vi "Download Bitfile.vi"(8 "error in (no error)":errorcluster, 10 "Port data.RIO device address":u16, 11 "path":path) -> (0 "error out":errorcluster, 5 "FPGA Session":u32)   [LabVIEW 2015, in "Diagnostics Addon Engine.lvlib"]
uses:
  Diagnostics Addon Engine.lvlib
  <vilib>/rvi/Utilities/XML/nirviXML_GetValue_String.vi
  NiFpga.dll
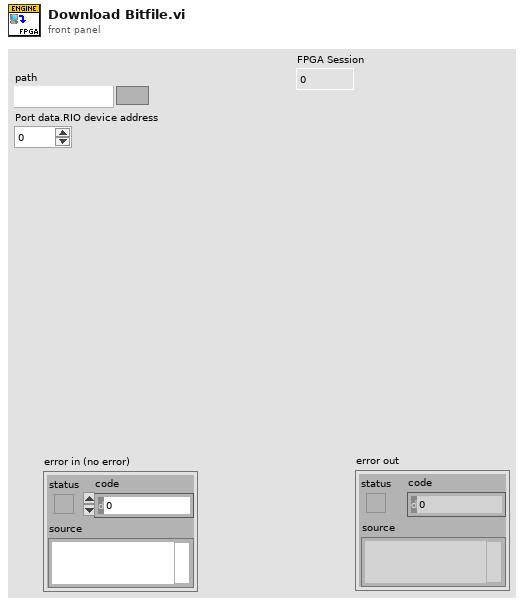
[diagram p1: front panel]
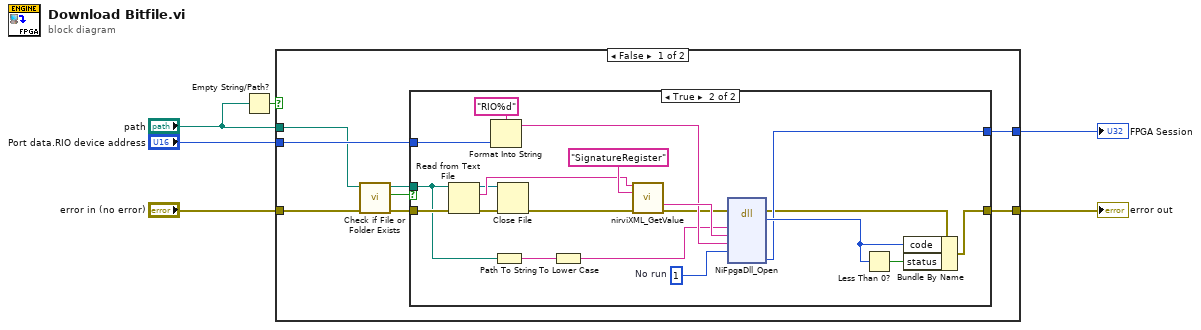
[diagram p0: block diagram]
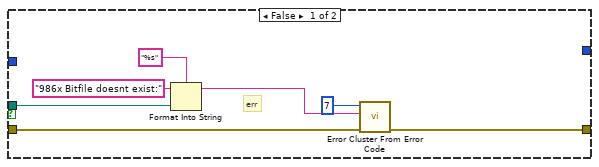
[diagram p2: hidden frame]
diagram:
  n1 = Empty String/Path?(string/path="path") -> (empty?=w3:bool)
  n2 = case shown="False" w3 {
    tunnel: "error in (no error)" -> [w13 w42]
    tunnel: [w14 w42] -> w5
    tunnel: "path" -> [w7 _]
    tunnel: "Port data.RIO device address" -> [w9 _]
    tunnel: [w8 _] -> w4
    frame False {
      n3 = call <vilib>:"Check if File or Folder Exists.vi"("error in (no error)"=w13, "path"=w7) -> ("error out"=w12:errorcluster, "file or folder exists?"=w11:bool, "dup path"=w10:path)  [unwired: 7 in]
      n4 = case shown="True" w11 {
        tunnel: [w16 w38] -> w14
        tunnel: w12 -> [w18 w31]
        tunnel: w10 -> [w21 w30]
        tunnel: w9 -> [_ w28]
        tunnel: [_ w26] -> w8
        frame False {
          # "err"
          n5 = Format Into String(format string="%s", initial string="986x Bitfile doesnt exist:", w21) -> (resulting string=w17:string)  [unwired: 1 in, 1 out]
          n6 = call <vilib>:"Error Cluster From Error Code.vi"("error in (no error)"=w18, "error message (\"\")"=w17, "error code (0)"=7) -> ("error out"=w16:errorcluster)  [unwired: 1 in, 5 out]
        }
        frame True {
          w37 = u32 1  # No run
          n7 = Read from Text File(file (use dialog)=w30, error in=w31) -> (refnum out=w34:refnum<file>, text=w35:string, error out=w33:errorcluster)  [unwired: 3 out]
          n8 = Format Into String(format string="RIO%d", w28) -> (resulting string=w27:string)  [unwired: 2 in, 1 out]
          n9 = Path To String(path=w30) -> (string=w41:string)
          n10 = Close File(refnum=w34, error in=w33) -> (error out=w32:errorcluster)  [unwired: 1 out]
          n11 = To Lower Case(string=w41) -> (all lower case string=w23:string)
          n12 = call-poly <vilib>:"nirviXML_GetValue.vi"("xml string in"=w35, "tag name in"="SignatureRegister" ("tag"), "error in (no error)"=w32) -> ("value"=w29:string, "error out"=w25:errorcluster)  [unwired: 2 in, 9 out]
          n13 = dll-call lib="NiFpga.*" fn="NiFpgaDll_Open"(error in=w25, "Bitfile"=w23, "Signature"=w29, "Resource"=w27, "Attribute"=w37) -> (error out=w24:errorcluster, "Status"=w39:i32, "Session"=w26:u32)  [unwired: 7 in, 1 out]
          n14 = Less Than 0?(x=w39) -> (x < 0?=w40:bool)
          n15 = Bundle By Name(cluster=w24, "code"=w39, "status"=w40) -> (w38:errorcluster)
        }
      }
    }
    frame True {
    }
  }
  "error out" <- w5
  "FPGA Session" <- w4
